vi "Convert Experiment Folder.vi"(8 "error in (no error)":errorcluster, 10 "Experiment Folder File Type":T1, 11 "Experiment Folder Path":path) -> (0 "error out":errorcluster)   [LabVIEW 2016, in "Conversion.lvclass"]
uses:
  Conversion.lvclass
  Data/Typedefs/File Type--enum.ctl
  <userlib>/_OpenG.lib/lvzip/lvzip.llb/ZLIB Zip Handle__ogtk.ctl
  Conversion.lvclass/Conversion.ctl
  <userlib>/_OpenG.lib/file/file.llb/Build Path - File Names Array__ogtk.vi
  <userlib>/_OpenG.lib/file/file.llb/Convert File Extension (Path)__ogtk.vi
  <userlib>/_OpenG.lib/file/file.llb/Compare Two Paths - Scalar__ogtk.vi
  <userlib>/_OpenG.lib/lvzip/lvzip.llb/ZLIB Store File__ogtk.vi
  Data/Data.lvclass
panel:
  out "File":string
  out "State":string
  in  "OK":bool
  in  "Additional Notes?":string
  out "Elapsed Time (s)":dbl
  out "Remaining Files":i32
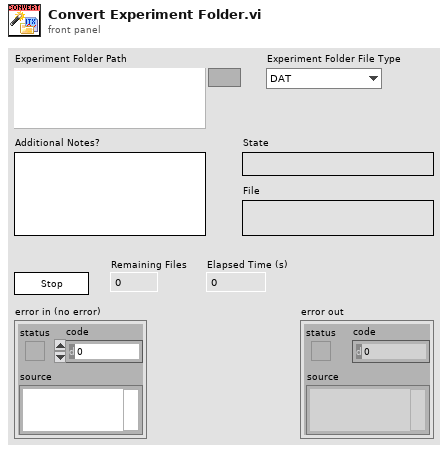
[diagram p1: front panel]
types:
  T1 = typedef "Data.lvclass/File Type--enum.ctl" = enum16{"DAT", "ITX", "TDMS", "VI", "PGSQL"}
  T2 = enum32{"Invalid", "Standard", "Closed", "Hidden", "Minimized", "Maximized"}
  T3 = enum32{"invalid app kind", "Development System", "Run Time System", "Student Edition", "Embedded LabVIEW", "Evaluation", "Custom"}
  T4 = typedef "ZLIB Zip Handle__ogtk.ctl" = refnum<k1>
  T5 = cluster{"Core":cluster{"Current VI Reference":refnum<vi>, "Close Panel on Exit?":bool}, "Conversion.lvclass":refnum<class "Conversion.lvclass">, "Experiment Folder Path":path, "Files to Zip":path[], "zip Refnum":T4, "Start Time":dbl, "Conversion End Time":dbl, "Archive End Time":dbl, "File Index":i32, "Number of Files":i32, "Log File Path":path}
  T6 = cluster{"Current VI Reference":refnum<vi>, "Close Panel on Exit?":bool}
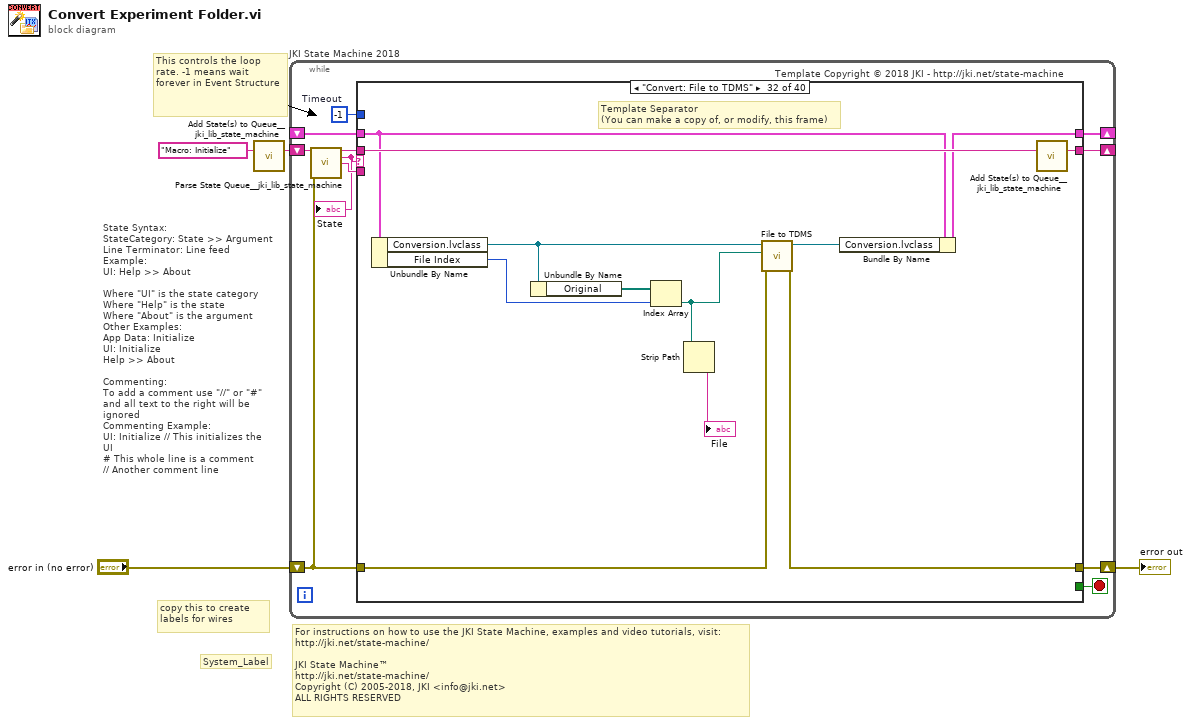
[diagram p0: block diagram]
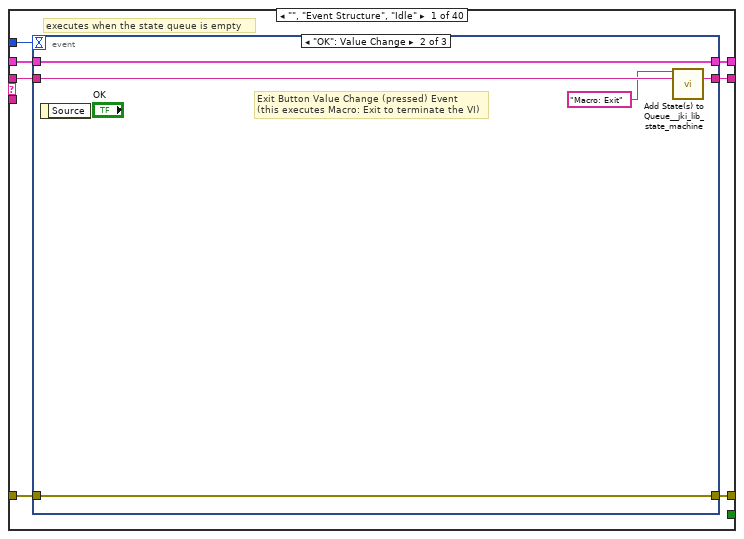
[diagram p2: hidden frame]
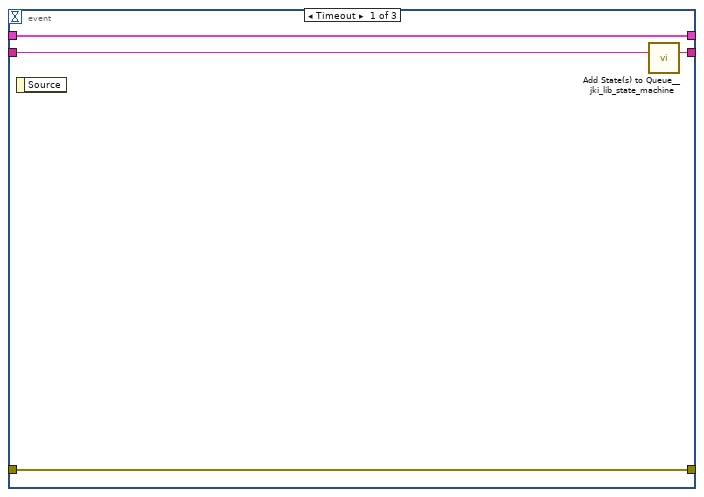
[diagram p3: hidden frame]
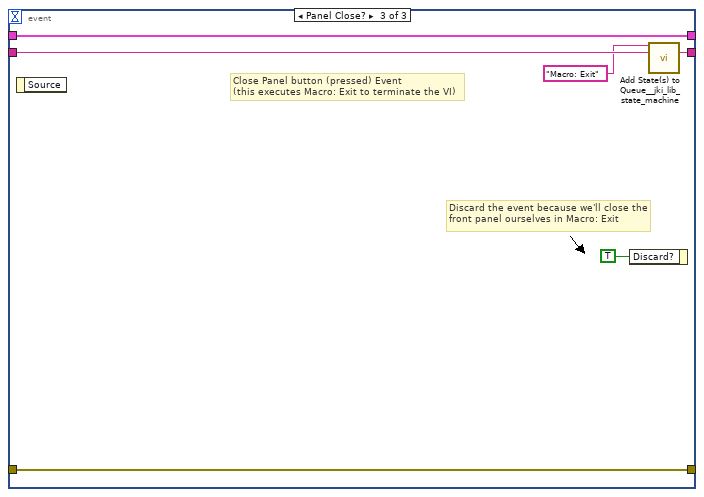
[diagram p4: hidden frame]
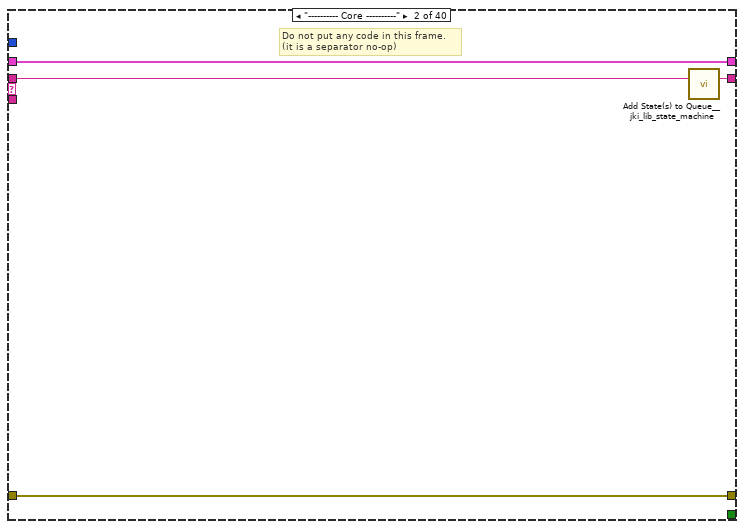
[diagram p5: hidden frame]
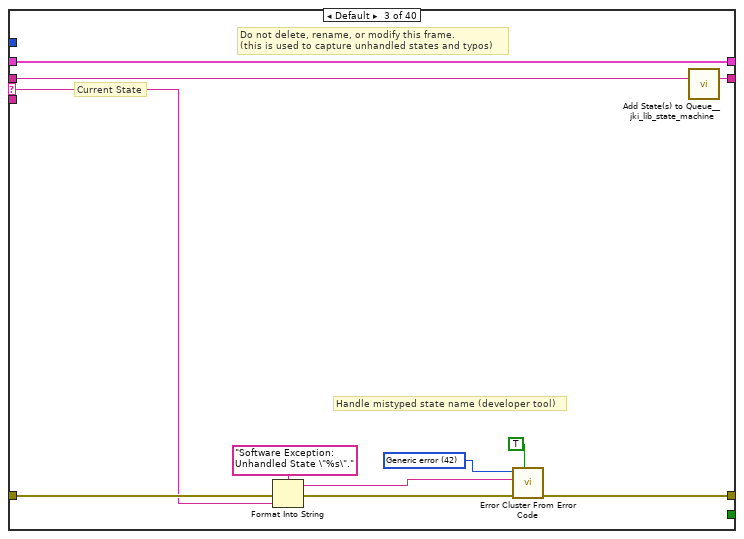
[diagram p6: hidden frame]
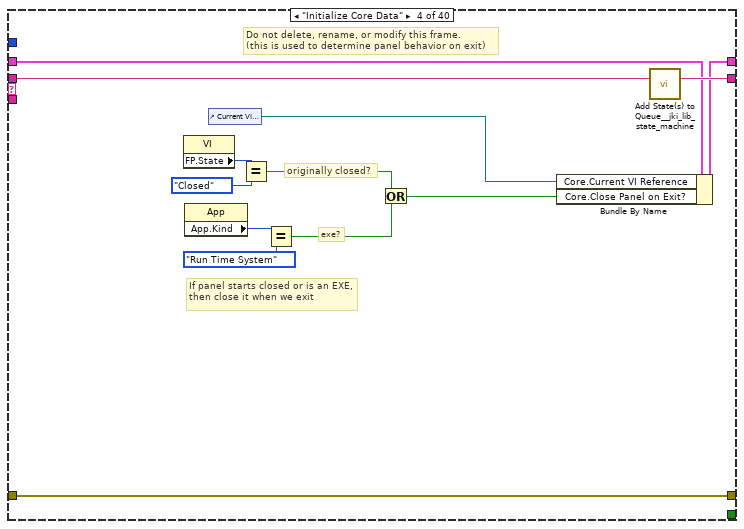
[diagram p7: hidden frame]
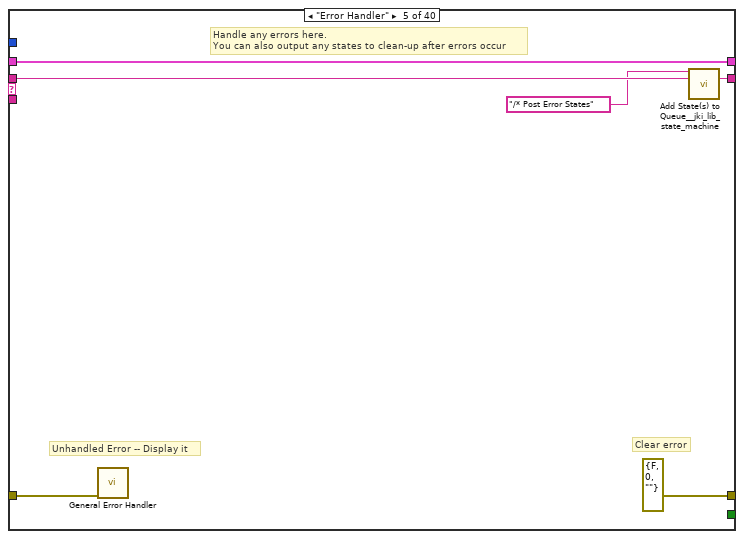
[diagram p8: hidden frame]
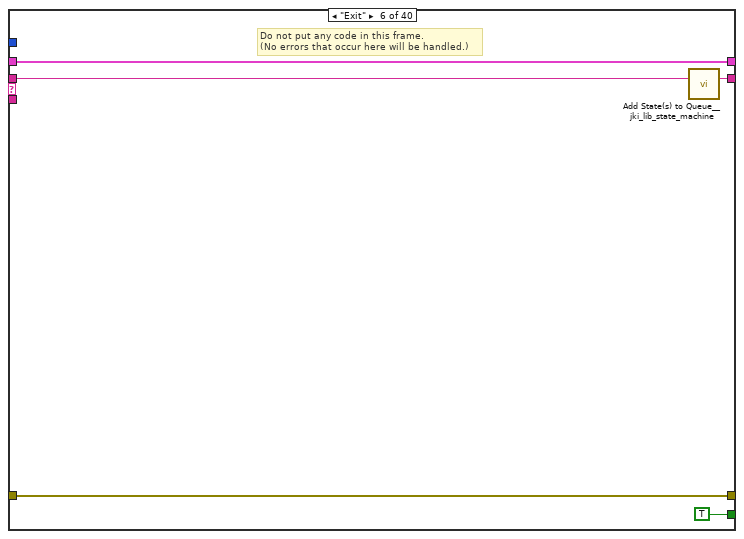
[diagram p9: hidden frame]
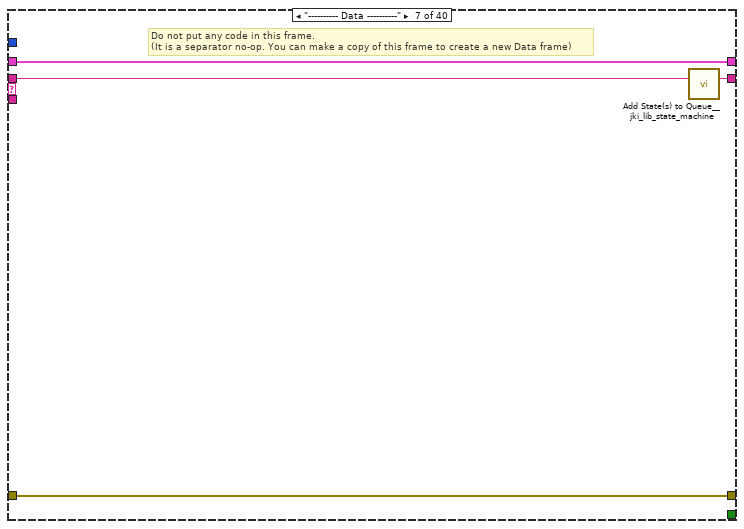
[diagram p10: hidden frame]
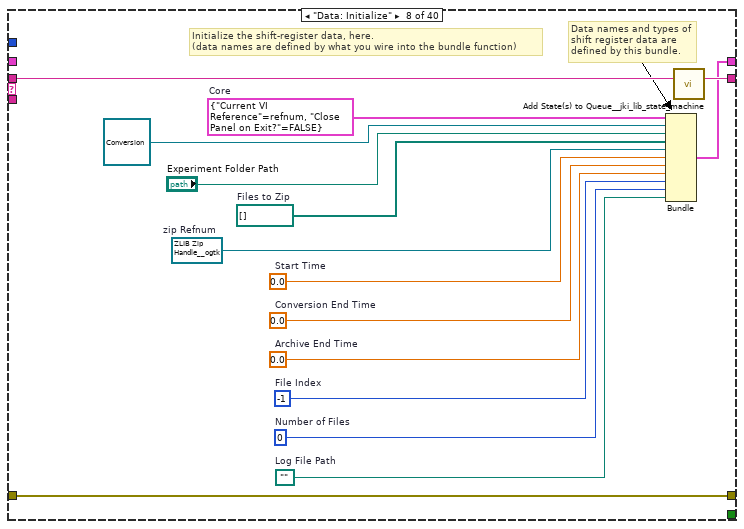
[diagram p11: hidden frame]
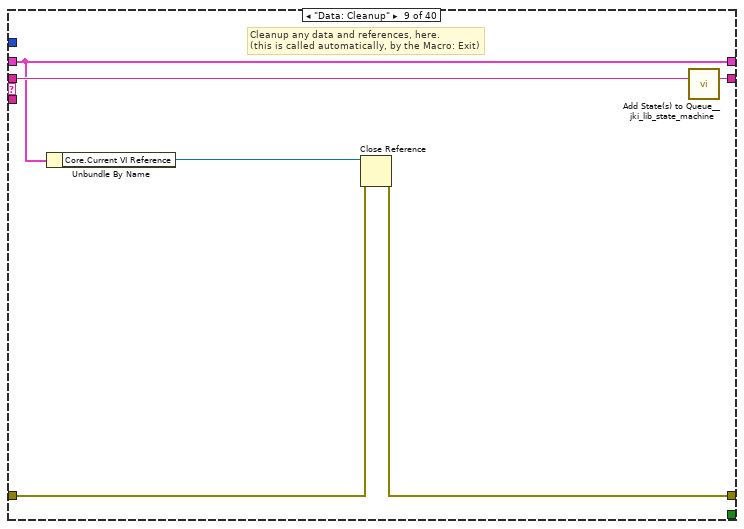
[diagram p12: hidden frame]
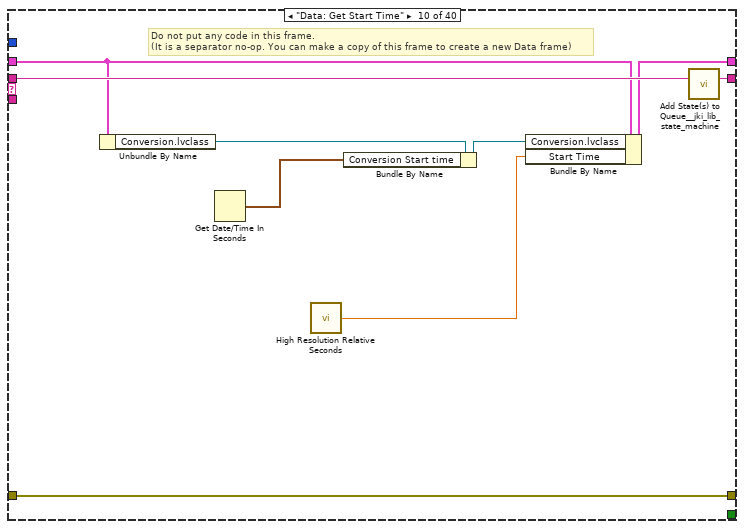
[diagram p13: hidden frame]
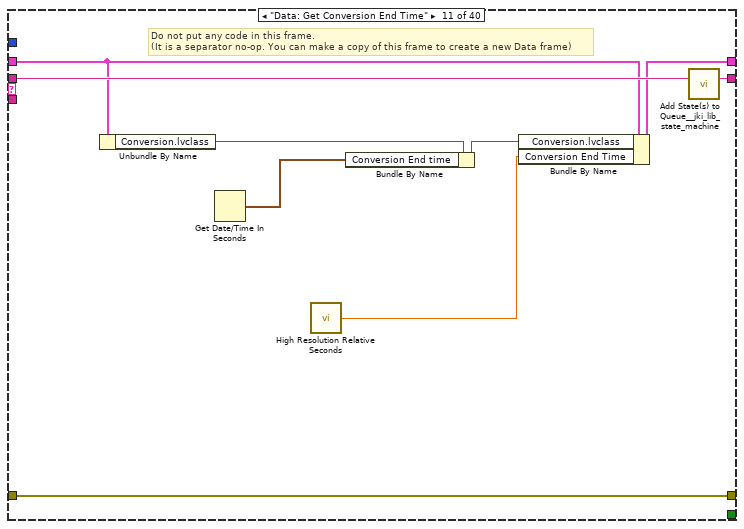
[diagram p14: hidden frame]
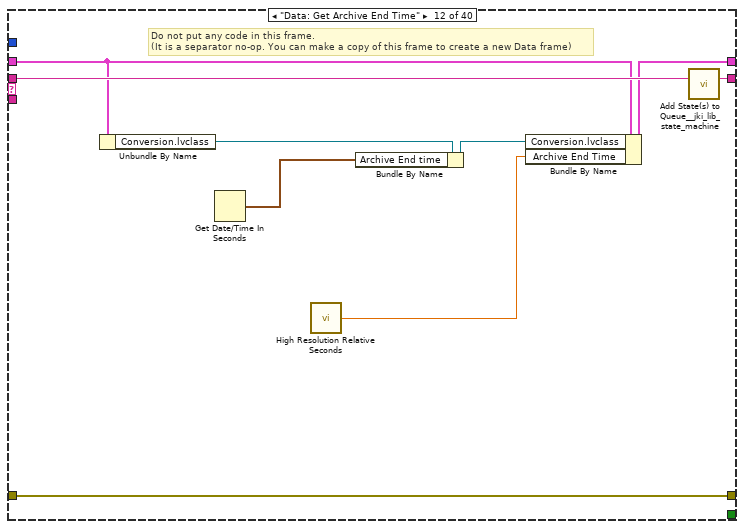
[diagram p15: hidden frame]
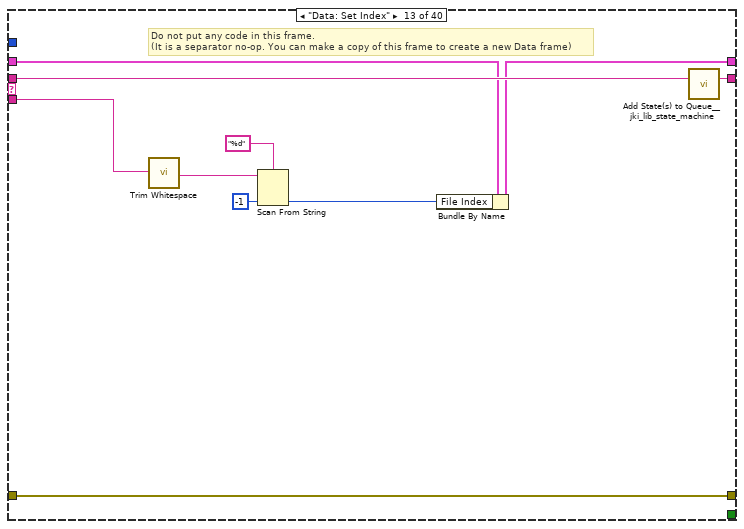
[diagram p16: hidden frame]
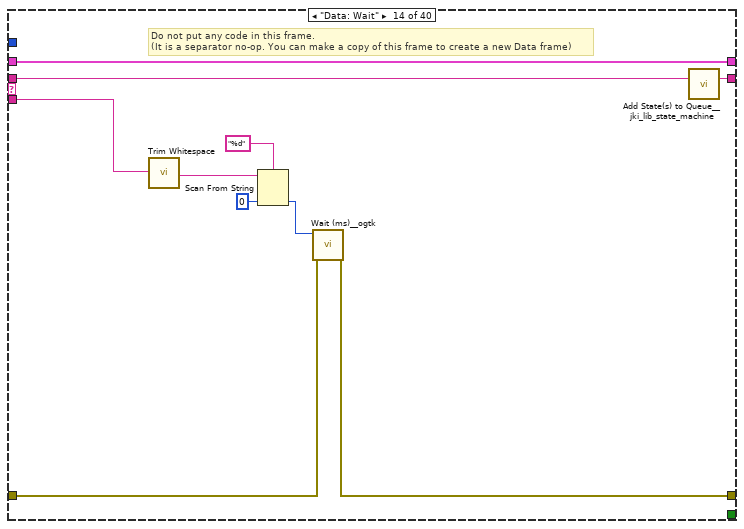
[diagram p17: hidden frame]
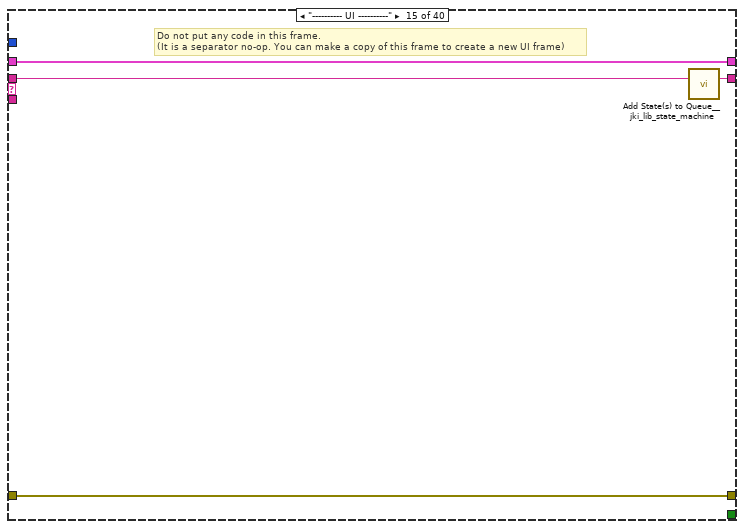
[diagram p18: hidden frame]
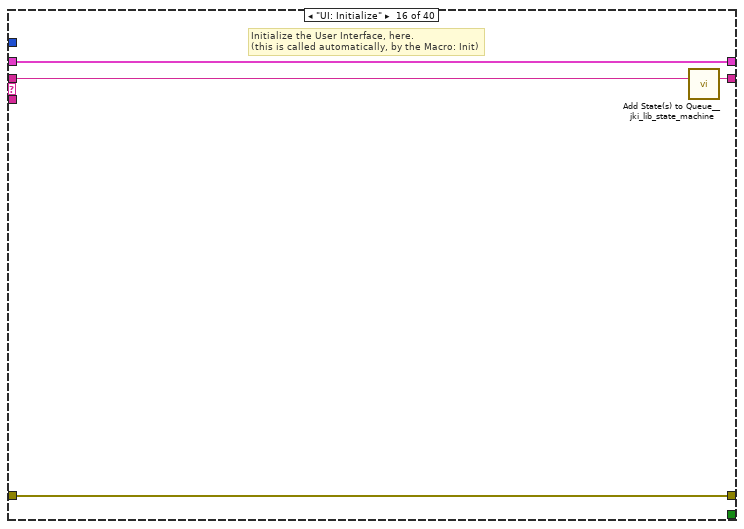
[diagram p19: hidden frame]
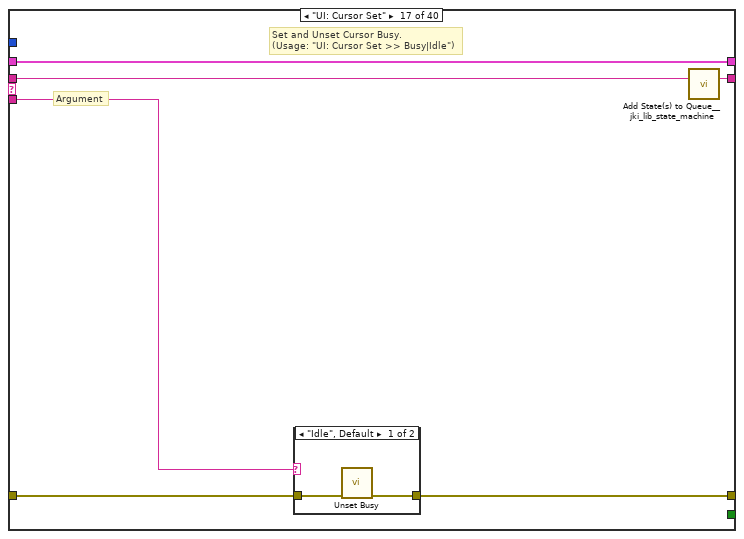
[diagram p20: hidden frame]
diagram:
  # "For instructions on how to use the JKI State Machine, examples and video tutorials, visit:\nhttp://jki.net/state-machine/\n\nJKI State Machine™\nhttp://jki.net/state-machine/\nCopyright (C) 2005-2018, JKI <info@jki.net>\nALL RIGHTS RESERVED"
  # "State Syntax:\nStateCategory: State >> Argument\nLine Terminator: Line feed\nExample:\nUI: Help >> About\n\nWhere \"UI\" is the state category\nWhere \"Help\" is the state\nWhere \"About\" is the argument\nOther Examples:\nApp Data: Initialize\nUI: Initialize\nHelp >> About\n\nCommenting:\nTo add a comment use \"//\" or \"#\" and all text to the right will be ignored\nCommenting Example:\nUI: Initialize // This initializes the UI\n# This whole line is a comment\n// Another comment line"
  # "copy this to create labels for wires"
  # "This controls the loop rate. -1 means wait forever in Event Structure"
  # "System_Label"
  n1 = call <vilib>:"Add State(s) to Queue__jki_lib_state_machine.vi"("State(s) in (\"\")"="Macro: Initialize") -> ("States Out"=w4:string)  [unwired: 14 in]
  n2 = while "JKI State Machine 2018" {
    shift-right: [w9] -> _
    shift-left: _ -> [w8]
    shift-right: [w12] -> w1
    shift-left: "error in (no error)" -> [w6]
    shift-right: [w11] -> _
    shift-left: w4 -> [w13]
    stop <- w10 stop-if-true
    w7 = -1  # Timeout
    # "Template Copyright © 2018 JKI - http://jki.net/state-machine"
    n3 = call <vilib>:"Parse State Queue__jki_lib_state_machine.vi"("State Queue"=w13, "Error In (no error)"=w6) -> ("Remaining States"=w15:string, "Current State"=w5:string, "Arguments"=w14:string)  [unwired: 11 in]
    "State" <- w5
    n4 = case shown="\"Convert: File to TDMS\"" w5 {
      selector: w5 -> [_ _ w42 _ _ _ _ _ _ _ _ _ _ _ _ _ _ _ _ _ _ _ _ _ _ _ _ _ _ _ _ _ _ _ _ _ _ _ _ _]
      tunnel: w15 -> [w22 w41 w46 w65 w71 w76 w80 w95 w101 w110 w119 w128 w138 w148 w152 w156 w162 w173 w245 w252 w256 w261 w266 w282 w287 w292 w307 w312 w322 w326 w341 w356 w368 w375 w385 w396 w401 w420 w437 w443]
      tunnel: w14 -> [_ _ _ _ _ _ _ _ _ _ _ _ w129 w142 _ _ w157 w167 _ _ _ _ _ _ _ _ _ _ _ _ _ _ _ _ _ _ _ _ _ _]
      tunnel: w8 -> [w20 w38 w44 w58 w68 w74 w77 _ w96 w107 w116 w125 w134 w146 w149 w154 w160 w169 w242 w249 w253 w258 w263 w270 w284 w289 w295 w309 w319 w323 w338 w351 w365 w371 w379 w392 w398 w413 w433 w440]
      tunnel: [w19 w39 w48 w62 errorcluster {"status"=FALSE, "code"=0, "source"=""} ("error out") w73 w78 w92 w97 w108 w117 w126 w136 w139 w150 w153 w158 w170 w243 w250 w254 w259 w264 w280 w285 w290 w305 w310 w320 w324 w333 w354 w360 w369 w381 w386 w399 w418 w428 w438] -> w12
      tunnel: w6 -> [w18 w39 w47 w62 w67 w73 w78 w92 w98 w108 w117 w126 w136 w140 w150 w153 w159 w171 w243 w250 w254 w259 w264 w280 w285 w290 w305 w310 w320 w324 w334 w345 w361 w370 w382 w387 w399 w409 w427 w439]
      tunnel: [w21 w40 w45 w64 w70 w75 w79 w94 w100 w109 w118 w127 w137 w147 w151 w155 w161 w172 w244 w251 w255 w260 w265 w281 w286 w291 w306 w311 w321 w325 w340 w355 w367 w374 w384 w395 w400 w419 w436 w442] -> w11
      tunnel: [_ _ _ _ _ TRUE _ _ _ _ _ _ _ _ _ _ _ _ _ _ _ _ _ _ _ _ _ _ _ _ _ _ _ _ _ _ _ _ _ _] -> w10
      tunnel: [w17 w38 w44 w63 w68 w74 w77 w93 w96 w106 w115 w124 w135 w146 w149 w154 w160 w169 w242 w249 w253 w258 w263 w270 w284 w289 w295 w309 w319 w323 w337 w350 w364 w371 w378 w392 w398 w412 w432 w440] -> w9
      tunnel: w7 -> [w16 _ _ _ _ _ _ _ _ _ _ _ _ _ _ _ _ _ _ _ _ _ _ _ _ _ _ _ _ _ _ _ _ _ _ _ _ _ _ _]
      frame "", "Event Structure", "Idle" {
        # "executes when the state queue is empty"
        n5 = event shown="[1] \"OK\": Value Change" {
          selector: _ -> [_ _ _]
          dyn-events: _ -> [_ _ _]
          timeout: w16 -> [_ _ _]
          tunnel: w22 -> [w26 w31 w37]
          tunnel: [w25 w30 w36] -> w21
          tunnel: w20 -> [w24 w28 w34]
          tunnel: [w23 w29 w35] -> w19
          tunnel: w18 -> [w23 w29 w35]
          tunnel: [w24 w28 w34] -> w17
          event Timeout {
            n6 = event-data() -> ()  [unwired: 1 in, 1 out]
            n7 = call <vilib>:"Add State(s) to Queue__jki_lib_state_machine.vi"("State(s) in (\"\")"=w26) -> ("States Out"=w25:string)  [unwired: 14 in]
          }
          event "OK": Value Change {
            # "Exit Button Value Change (pressed) Event\n(this executes Macro: Exit to terminate the VI)"
            n8 = event-data() -> ()  [unwired: 1 in, 1 out]
            n9 = call <vilib>:"Add State(s) to Queue__jki_lib_state_machine.vi"("State(s) in Front (\"\")"="Macro: Exit", "State(s) in (\"\")"=w31) -> ("States Out"=w30:string)  [unwired: 13 in]
          }
          event Panel Close? {
            # "Discard the event because we'll close the front panel ourselves in Macro: Exit"
            # "Close Panel button (pressed) Event\n(this executes Macro: Exit to terminate the VI)"
            n10 = event-data() -> ()  [unwired: 1 in, 1 out]
            n11 = event-data("Discard?"=TRUE) -> ()  [unwired: 1 in, 1 out]
            n12 = call <vilib>:"Add State(s) to Queue__jki_lib_state_machine.vi"("State(s) in Front (\"\")"="Macro: Exit", "State(s) in (\"\")"=w37) -> ("States Out"=w36:string)  [unwired: 13 in]
          }
        }
      }
      frame "---------- Core ----------" {
        # "Do not put any code in this frame.\n(it is a separator no-op)"
        n13 = call <vilib>:"Add State(s) to Queue__jki_lib_state_machine.vi"("State(s) in (\"\")"=w41) -> ("States Out"=w40:string)  [unwired: 14 in]
      }
      frame Default {
        w51 = 42 items=["No error", "Argument error", "Memory is full", "Out of zone", "End of file", "File already open", "Generic file I/O error", "File not found", "File permission error", "Disk is full", "Duplicate path", "Too many files open", "System feature not enabled", "Resource file not found", "Cannot add resource", "Resource not found", "Image not found", "Image memory error", "Pen does not exist", "Config type invalid", "Config token not found", "Config parse error", "Config memory error", "Bad external code format", "Bad external code offset", "External code not present", "Null window", "Destroy window error", "Null menu", "Print aborted", "Bad print record", "Print driver error", "Windows error during printing", "Memory error during printing", "Print dialog error", "Generic print error", "Invalid device refnum", "Device not found", "Device parameter error", "Device unit error", "Cannot open device", "Device call aborted", "Generic error", "Cancelled by user", "Object ID too low", "Object ID too high", "Object not in heap", "Unknown heap", "Unknown object (invalid DefProc)", "Unknown object (DefProc not in table)", "Message out of range", "Invalid (null) method", "Unknown message", "Manager call not supported", "Bad address", "Network operation in progress", "Network operation timed out", "Connection is busy", "Network attribute not supported", "Network error", "Address in use", "System out of memory", "Connection aborted", "Connection refused", "Not connected", "Already connected", "Connection closed", "Initialization error (interapplication manager)", "Bad occurrence", "Wait on unbound occurrence handler", "Occurrence queue overflow", "Datalog type conflict", "Unused", "Unrecognized type (interapplication manager)", "Memory corrupt", "Failed to make temporary DLL", "Old CIN version", "Drag socket not found", "Failed to load drop-object", "Failed to register OLE object", "Failed to release OLE object", "Format specifier type mismatch", "Unknown format specifier", "Too few format specifiers", "Too many format specifiers", "Scan failed", "Newer CIN version", "Error converting to variant", "Runtime menu error", "Password tampered", "Variant attribute not found", "Incompatible variant data type", "Event data is not available", "Event Store is not present", "Occurrence is not found", "Event Queue is not created", "Event info is not available", "Refnum passed is NULL", "Error retrieving Class GUID", "Error retrieving CoClass GUID", "Error retrieving TypeLib GUID.", "Bad built application magic bytes.", "Specific driver is different from the specific driver associated with the Logical Name.", "There is no session opened to the class driver.", "Max Error", "MAX - Error with config objects", "MAX - Error loading configuration", "MAX - Group not supported"]
        # "Current State"
        # "Do not delete, rename, or modify this frame.\n(this is used to capture unhandled states and typos)"
        # "Handle mistyped state name (developer tool)"
        n14 = Format Into String(format string="Software Exception: Unhandled State \"%s\"." ("message"), error in=w47, w42) -> (resulting string=w50:string, error out=w49:errorcluster)  [unwired: 1 in]
        n15 = call <vilib>:"Error Cluster From Error Code.vi"("show call chain? (False)"=TRUE, "error in (no error)"=w49, "error message (\"\")"=w50, "error code (0)"=w51) -> ("error out"=w48:errorcluster)  [unwired: 5 in]
        n16 = call <vilib>:"Add State(s) to Queue__jki_lib_state_machine.vi"("State(s) in (\"\")"=w46) -> ("States Out"=w45:string)  [unwired: 14 in]
      }
      frame "Initialize Core Data" {
        # "Do not delete, rename, or modify this frame.\n(this is used to determine panel behavior on exit)"
        # "originally closed?"
        # "exe?"
        # "If panel starts closed or is an EXE, then close it when we exit"
        n17 = property class="VI"() -> ("FP.State"=w55:T2)  [unwired: 2 in, 2 out]
        n18 = property class="App"() -> ("App.Kind"=w61:T3)  [unwired: 2 in, 2 out]
        n19 = control-ref of="Current VI Reference"() -> (w56:refnum<vi>)
        n20 = Equal?(x=w55, y=T2."Closed" ("Front Panel Window:State")) -> (x = y?=w53:bool)
        n21 = Equal?(x=w61, y=T3."Run Time System" ("Application:Kind")) -> (x = y?=w59:bool)
        n22 = Or(x=w53, y=w59) -> (x .or. y?=w57:bool)
        n23 = Bundle By Name(cluster=w58, "Core.Current VI Reference"=w56, "Core.Close Panel on Exit?"=w57) -> (w63:T5)
        n24 = call <vilib>:"Add State(s) to Queue__jki_lib_state_machine.vi"("State(s) in (\"\")"=w65) -> ("States Out"=w64:string)  [unwired: 14 in]
      }
      frame "Error Handler" {
        # "Unhandled Error -- Display it"
        # "Handle any errors here.\nYou can also output any states to clean-up after errors occur"
        # "Clear error"
        n25 = call <vilib>:"General Error Handler.vi"("error in (no error)"=w67) -> ()  [unwired: 10 in, 5 out]
        n26 = call <vilib>:"Add State(s) to Queue__jki_lib_state_machine.vi"("State(s) in Front (\"\")"="/* Post Error States", "State(s) in (\"\")"=w71) -> ("States Out"=w70:string)  [unwired: 13 in]
      }
      frame "Exit" {
        # "Do not put any code in this frame.\n(No errors that occur here will be handled.)"
        n27 = call <vilib>:"Add State(s) to Queue__jki_lib_state_machine.vi"("State(s) in (\"\")"=w76) -> ("States Out"=w75:string)  [unwired: 14 in]
      }
      frame "---------- Data ----------" {
        # "Do not put any code in this frame.\n(It is a separator no-op. You can make a copy of this frame to create a new Data frame)"
        n28 = call <vilib>:"Add State(s) to Queue__jki_lib_state_machine.vi"("State(s) in (\"\")"=w80) -> ("States Out"=w79:string)  [unwired: 14 in]
      }
      frame "Data: Initialize" {
        w81 = path[] []  # Files to Zip
        w82 = T4 refnum items=["zip"]  # zip Refnum
        w85 = 0.0  # Archive End Time
        w86 = path ""  # Log File Path
        w87 = 0  # Number of Files
        w88 = -1  # File Index
        w89 = 0.0  # Conversion End Time
        w90 = 0.0  # Start Time
        w91 = T6 {"Current VI Reference"=refnum, "Close Panel on Exit?"=FALSE}  # Core
        # "Data names and types of shift register data are defined by this bundle."
        # "Initialize the shift-register data, here.\n(data names are defined by what you wire into the bundle function)"
        n29 = Bundle("Core"=w91, "Conversion.lvclass"=refnum<class "Conversion.lvclass"> refnum, "Experiment Folder Path"="Experiment Folder Path", "Files to Zip"=w81, "zip Refnum"=w82, "Start Time"=w90, "Conversion End Time"=w89, "Archive End Time"=w85, "File Index"=w88, "Number of Files"=w87, "Log File Path"=w86) -> (w93:T5)  [unwired: 1 in]
        n30 = call <vilib>:"Add State(s) to Queue__jki_lib_state_machine.vi"("State(s) in (\"\")"=w95) -> ("States Out"=w94:string)  [unwired: 14 in]
      }
      frame "Data: Cleanup" {
        # "Cleanup any data and references, here.\n(this is called automatically, by the Macro: Exit)"
        n31 = Unbundle By Name(w96) -> ("Core.Current VI Reference"=w99:refnum<vi>)
        n32 = Close Reference(reference=w99, error in (no error)=w98) -> (error out=w97:errorcluster)
        n33 = call <vilib>:"Add State(s) to Queue__jki_lib_state_machine.vi"("State(s) in (\"\")"=w101) -> ("States Out"=w100:string)  [unwired: 14 in]
      }
      frame "Data: Get Start Time" {
        # "Do not put any code in this frame.\n(It is a separator no-op. You can make a copy of this frame to create a new Data frame)"
        n34 = Unbundle By Name(w107) -> ("Conversion.lvclass"=w104:refnum<class "Conversion.lvclass">)
        n35 = Get Date/Time In Seconds() -> (seconds since 1Jan1904=w105:timestamp)
        n36 = call <vilib>:"High Resolution Relative Seconds.vi"() -> ("relative seconds"=w102:dbl)
        n37 = Bundle By Name(cluster=w104, "Conversion Start time"=w105) -> (w103:refnum<class "Conversion.lvclass">)
        n38 = Bundle By Name(cluster=w107, "Conversion.lvclass"=w103, "Start Time"=w102) -> (w106:T5)
        n39 = call <vilib>:"Add State(s) to Queue__jki_lib_state_machine.vi"("State(s) in (\"\")"=w110) -> ("States Out"=w109:string)  [unwired: 14 in]
      }
      frame "Data: Get Conversion End Time" {
        # "Do not put any code in this frame.\n(It is a separator no-op. You can make a copy of this frame to create a new Data frame)"
        n40 = Unbundle By Name(w116) -> ("Conversion.lvclass"=w113:refnum<class "Conversion.lvclass">)
        n41 = Get Date/Time In Seconds() -> (seconds since 1Jan1904=w114:timestamp)
        n42 = call <vilib>:"High Resolution Relative Seconds.vi"() -> ("relative seconds"=w111:dbl)
        n43 = Bundle By Name(cluster=w113, "Conversion End time"=w114) -> (w112:refnum<class "Conversion.lvclass">)
        n44 = Bundle By Name(cluster=w116, "Conversion.lvclass"=w112, "Conversion End Time"=w111) -> (w115:T5)
        n45 = call <vilib>:"Add State(s) to Queue__jki_lib_state_machine.vi"("State(s) in (\"\")"=w119) -> ("States Out"=w118:string)  [unwired: 14 in]
      }
      frame "Data: Get Archive End Time" {
        # "Do not put any code in this frame.\n(It is a separator no-op. You can make a copy of this frame to create a new Data frame)"
        n46 = Unbundle By Name(w125) -> ("Conversion.lvclass"=w122:refnum<class "Conversion.lvclass">)
        n47 = Get Date/Time In Seconds() -> (seconds since 1Jan1904=w123:timestamp)
        n48 = call <vilib>:"High Resolution Relative Seconds.vi"() -> ("relative seconds"=w120:dbl)
        n49 = Bundle By Name(cluster=w122, "Archive End time"=w123) -> (w121:refnum<class "Conversion.lvclass">)
        n50 = Bundle By Name(cluster=w125, "Conversion.lvclass"=w121, "Archive End Time"=w120) -> (w124:T5)
        n51 = call <vilib>:"Add State(s) to Queue__jki_lib_state_machine.vi"("State(s) in (\"\")"=w128) -> ("States Out"=w127:string)  [unwired: 14 in]
      }
      frame "Data: Set Index" {
        # "Do not put any code in this frame.\n(It is a separator no-op. You can make a copy of this frame to create a new Data frame)"
        n52 = call <vilib>:"Trim Whitespace.vi"("string"=w129) -> ("trimmed string"=w133:string)  [unwired: 1 in]
        n53 = Scan From String(format string="%d", input string=w133, default 1=-1 ("default value 1")) -> (output 1=w130:i32)  [unwired: 2 in, 3 out]
        n54 = Bundle By Name(cluster=w134, "File Index"=w130) -> (w135:T5)
        n55 = call <vilib>:"Add State(s) to Queue__jki_lib_state_machine.vi"("State(s) in (\"\")"=w138) -> ("States Out"=w137:string)  [unwired: 14 in]
      }
      frame "Data: Wait" {
        # "Do not put any code in this frame.\n(It is a separator no-op. You can make a copy of this frame to create a new Data frame)"
        n56 = call <vilib>:"Trim Whitespace.vi"("string"=w142) -> ("trimmed string"=w145:string)  [unwired: 1 in]
        n57 = Scan From String(format string="%d", input string=w145, default 1=0 ("default value 1")) -> (output 1=w141:i32)  [unwired: 2 in, 3 out]
        n58 = call <userlib>:"Wait (ms)__ogtk.vi"("error in (no error)"=w140, "milliseconds to wait"=w141) -> ("error out"=w139:errorcluster)  [unwired: 8 in, 1 out]
        n59 = call <vilib>:"Add State(s) to Queue__jki_lib_state_machine.vi"("State(s) in (\"\")"=w148) -> ("States Out"=w147:string)  [unwired: 14 in]
      }
      frame "---------- UI ----------" {
        # "Do not put any code in this frame.\n(It is a separator no-op. You can make a copy of this frame to create a new UI frame)"
        n60 = call <vilib>:"Add State(s) to Queue__jki_lib_state_machine.vi"("State(s) in (\"\")"=w152) -> ("States Out"=w151:string)  [unwired: 14 in]
      }
      frame "UI: Initialize" {
        # "Initialize the User Interface, here.\n(this is called automatically, by the Macro: Init)"
        n61 = call <vilib>:"Add State(s) to Queue__jki_lib_state_machine.vi"("State(s) in (\"\")"=w156) -> ("States Out"=w155:string)  [unwired: 14 in]
      }
      frame "UI: Cursor Set" {
        # "Argument"
        # "Set and Unset Cursor Busy.\n(Usage: \"UI: Cursor Set >> Busy|Idle\")"
        n62 = case shown="\"Idle\", Default" w157 {
          tunnel: w159 -> [w164 w166]
          tunnel: [w163 w165] -> w158
          frame "Idle", Default {
            n63 = call <vilib>:"Unset Busy.vi"("error in (no error)"=w164) -> ("error out"=w163:errorcluster)  [unwired: 10 in]
          }
          frame "Busy" {
            n64 = call <vilib>:"Set Busy.vi"("error in (no error)"=w166) -> ("error out"=w165:errorcluster)  [unwired: 9 in, 1 out]
          }
        }
        n65 = call <vilib>:"Add State(s) to Queue__jki_lib_state_machine.vi"("State(s) in (\"\")"=w162) -> ("States Out"=w161:string)  [unwired: 14 in]
      }
      frame "UI: Front Panel State" {
        # "Argument"
        # "Set Front Panel Open or Closed\n(Usage: \"UI: Front Panel State >> Open|Close\")"
        n66 = Unbundle By Name(w169) -> ("Core.Current VI Reference"=w168:refnum<vi>)
        n67 = case shown="\"Open\", \"Standard\", Default" w167 {
          tunnel: w171 -> [w179 w194 w205 w218 w231]
          tunnel: [w181 w195 w207 w220 w233] -> w170
          tunnel: w168 -> [w180 w192 w206 w219 w232]
          frame "Open", "Standard", Default {
            w174 = T2."Standard" ("State")
            n68 = property class="VI"(reference=w180, error in=w179) -> (reference out=w177:refnum<vi>, error out=w178:errorcluster, "FP.State"=w176:T2)
            n69 = Not Equal?(x=w176, y=w174) -> (x != y?=w175:bool)
            n70 = case shown="False" w175 {
              tunnel: [w185 w187] -> w181
              tunnel: w178 -> [w184 w187]
              tunnel: w177 -> [w183 _]
              tunnel: w174 -> [w182 _]
              frame True {
                n71 = invoke class="VI" method="FP.Open"(reference=w183, error in=w184, "Activate"=TRUE, "State"=w182) -> (error out=w185:errorcluster)  [unwired: 1 in, 4 out]
              }
              frame False {
              }
            }
          }
          frame "Close", "Closed" {
            n72 = property class="VI"(reference=w192, error in=w194) -> (reference out=w191:refnum<vi>, error out=w193:errorcluster, "FP.State"=w189:T2)
            n73 = Not Equal?(x=w189, y=T2."Closed" ("Front Panel Window:State")) -> (x != y?=w188:bool)
            n74 = case shown="True" w188 {
              tunnel: [w196 w199] -> w195
              tunnel: w193 -> [w196 w198]
              tunnel: w191 -> [_ w197]
              frame False {
              }
              frame True {
                n75 = invoke class="VI" method="FP.Close"(reference=w197, error in=w198) -> (error out=w199:errorcluster)  [unwired: 1 in, 2 out]
              }
            }
          }
          frame "Hidden", "Hide" {
            w200 = T2."Hidden" ("State")
            n76 = property class="VI"(reference=w206, error in=w205) -> (reference out=w203:refnum<vi>, error out=w204:errorcluster, "FP.State"=w202:T2)
            n77 = Not Equal?(x=w202, y=w200) -> (x != y?=w201:bool)
            n78 = case shown="True" w201 {
              tunnel: [w211 w212] -> w207
              tunnel: w204 -> [w210 w212]
              tunnel: w203 -> [w209 _]
              tunnel: w200 -> [w208 _]
              frame True {
                n79 = invoke class="VI" method="FP.Open"(reference=w209, error in=w210, "State"=w208) -> (error out=w211:errorcluster)  [unwired: 2 in, 4 out]
              }
              frame False {
              }
            }
          }
          frame "Minimize", "Minimized" {
            w213 = T2."Minimized" ("State")
            n80 = property class="VI"(reference=w219, error in=w218) -> (reference out=w216:refnum<vi>, error out=w217:errorcluster, "FP.State"=w215:T2)
            n81 = Not Equal?(x=w215, y=w213) -> (x != y?=w214:bool)
            n82 = case shown="True" w214 {
              tunnel: [w224 w225] -> w220
              tunnel: w217 -> [w223 w225]
              tunnel: w216 -> [w222 _]
              tunnel: w213 -> [w221 _]
              frame True {
                n83 = invoke class="VI" method="FP.Open"(reference=w222, error in=w223, "State"=w221) -> (error out=w224:errorcluster)  [unwired: 2 in, 4 out]
              }
              frame False {
              }
            }
          }
          frame "Maximize", "Maximized" {
            w226 = T2."Maximized" ("State")
            n84 = property class="VI"(reference=w232, error in=w231) -> (reference out=w229:refnum<vi>, error out=w230:errorcluster, "FP.State"=w228:T2)
            n85 = Not Equal?(x=w228, y=w226) -> (x != y?=w227:bool)
            n86 = case shown="True" w227 {
              tunnel: [w237 w238] -> w233
              tunnel: w230 -> [w236 w238]
              tunnel: w229 -> [w235 _]
              tunnel: w226 -> [w234 _]
              frame True {
                n87 = invoke class="VI" method="FP.Open"(reference=w235, error in=w236, "State"=w234) -> (error out=w237:errorcluster)  [unwired: 2 in, 4 out]
              }
              frame False {
              }
            }
          }
        }
        n88 = call <vilib>:"Add State(s) to Queue__jki_lib_state_machine.vi"("State(s) in (\"\")"=w173) -> ("States Out"=w172:string)  [unwired: 14 in]
      }
      frame "UI: Update Elapsed Time" {
        # "Do not put any code in this frame.\n(It is a separator no-op. You can make a copy of this frame to create a new UI frame)"
        n89 = Unbundle By Name(w242) -> ("Start Time"=w241:dbl)
        n90 = call <vilib>:"High Resolution Relative Seconds.vi"() -> ("relative seconds"=w240:dbl)
        n91 = Subtract(x=w240, y=w241) -> (x-y=→"Elapsed Time (s)":dbl)
        n92 = call <vilib>:"Add State(s) to Queue__jki_lib_state_machine.vi"("State(s) in (\"\")"=w245) -> ("States Out"=w244:string)  [unwired: 14 in]
      }
      frame "UI: Update Index" {
        # "Do not put any code in this frame.\n(It is a separator no-op. You can make a copy of this frame to create a new UI frame)"
        n93 = Unbundle By Name(w249) -> ("Number of Files"=w248:i32, "File Index"=w247:i32)
        n94 = Subtract(x=w248, y=w247) -> (x-y=→"Remaining Files":i32)
        n95 = call <vilib>:"Add State(s) to Queue__jki_lib_state_machine.vi"("State(s) in (\"\")"=w252) -> ("States Out"=w251:string)  [unwired: 14 in]
      }
      frame "---------- Macro ----------" {
        # "Do not put any code in this frame.\n(It is a separator no-op. You can make a copy of this frame to create a new Macro frame)"
        n96 = call <vilib>:"Add State(s) to Queue__jki_lib_state_machine.vi"("State(s) in (\"\")"=w256) -> ("States Out"=w255:string)  [unwired: 14 in]
      }
      frame "Macro: Initialize" {
        w257 = "Data: Initialize\nInitialize Core Data\nUI: Initialize\nUI: Front Panel State >> Open\nMacro: Convert Initialize\nMacro: Convert\nMacro: Zip Initialize\nMacro: Zip\nConvert: Write Log File\nConvert: Display Error\nMacro: Exit"  # Data: Initialize Initialize Core Data UI: Initialize UI: Front Panel State >> Open Macro: Convert Initialize Macro: Convert Macro: Zip Initialize Macro: Zip Convert: Write Log File Convert: Display Error Macro: Exit
        # "Initialization Macro\n(This is called once, when the VI starts)"
        n97 = call <vilib>:"Add State(s) to Queue__jki_lib_state_machine.vi"("State(s) in Front (\"\")"=w257, "State(s) in (\"\")"=w261) -> ("States Out"=w260:string)  [unwired: 13 in]
      }
      frame "Macro: Convert Initialize" {
        # "Initialization Macro\n(This is called once, when the VI starts)"
        n98 = call <vilib>:"Add State(s) to Queue__jki_lib_state_machine.vi"("State(s) in Front (\"\")"="\nData: Set Index >> -1\nConvert: Get Files\nData: Get Start Time\nUI: Update Index\nUI: Update Elapsed Time", "State(s) in (\"\")"=w266) -> ("States Out"=w265:string)  [unwired: 13 in]
      }
      frame "Macro: Convert" {
        # "Still Running?\n(OR are we done?)"
        # "next step"
        # "Initialization Macro\n(This is called once, when the VI starts)"
        n99 = Unbundle By Name(w270) -> ("File Index"=w274:i32, "Conversion.lvclass"=w269:refnum<class "Conversion.lvclass">)
        n100 = Unbundle By Name(w269) -> ("Original"=w268:path[])
        n101 = Increment(x=w274) -> (x+1=w271:i32)
        n102 = Array Size(array=w268) -> (size(s)=w278:i32)
        n103 = Decrement(x=w278) -> (x-1=w279:i32)
        n104 = In Range and Coerce(upper limit=w279, x=w271, lower limit=0) -> (In Range?=w276:bool)  [unwired: 1 out]
        n105 = Format Into String(format string="Data: Set Index >> %d\nUI: Update Index\nUI: Update Elapsed Time\nConvert: File to TDMS\n//\nMacro: Convert", w271) -> (resulting string=w273:string)  [unwired: 2 in, 1 out]
        n106 = Select(t=w273, s=w276, f="Macro: Convert Cleanup ") -> (s? t:f=w267:string)
        n107 = call <vilib>:"Add State(s) to Queue__jki_lib_state_machine.vi"("State(s) in Front (\"\")"=w267, "State(s) in (\"\")"=w282) -> ("States Out"=w281:string)  [unwired: 13 in]
      }
      frame "Macro: Convert Cleanup" {
        # "Initialization Macro\n(This is called once, when the VI starts)"
        n108 = call <vilib>:"Add State(s) to Queue__jki_lib_state_machine.vi"("State(s) in Front (\"\")"="Convert: Close File\nData: Get Conversion End Time\nUI: Update Elapsed Time", "State(s) in (\"\")"=w287) -> ("States Out"=w286:string)  [unwired: 13 in]
      }
      frame "Macro: Zip Initialize" {
        # "Do not put any code in this frame.\n(It is a separator no-op. You can make a copy of this frame to create a new Macro frame)"
        n109 = call <vilib>:"Add State(s) to Queue__jki_lib_state_machine.vi"("State(s) in Front (\"\")"="\nData: Set Index >> -1\nZip: Open\nUI: Update Elapsed Time", "State(s) in (\"\")"=w292) -> ("States Out"=w291:string)  [unwired: 13 in]
      }
      frame "Macro: Zip" {
        # "Still Running?\n(OR are we done?)"
        # "next step"
        # "Do not put any code in this frame.\n(It is a separator no-op. You can make a copy of this frame to create a new Macro frame)"
        n110 = Unbundle By Name(w295) -> ("File Index"=w299:i32, "Files to Zip"=w293:path[])
        n111 = Increment(x=w299) -> (x+1=w296:i32)
        n112 = Array Size(array=w293) -> (size(s)=w303:i32)
        n113 = Decrement(x=w303) -> (x-1=w304:i32)
        n114 = In Range and Coerce(upper limit=w304, x=w296, lower limit=0) -> (In Range?=w301:bool)  [unwired: 1 out]
        n115 = Format Into String(format string="Data: Set Index >> %d\nUI: Update Index\nUI: Update Elapsed Time\nZip: Add File\n//\nMacro: Zip", w296) -> (resulting string=w298:string)  [unwired: 2 in, 1 out]
        n116 = Select(t=w298, s=w301, f="Macro: Zip Cleanup") -> (s? t:f=w294:string)
        n117 = call <vilib>:"Add State(s) to Queue__jki_lib_state_machine.vi"("State(s) in Front (\"\")"=w294, "State(s) in (\"\")"=w307) -> ("States Out"=w306:string)  [unwired: 13 in]
      }
      frame "Macro: Zip Cleanup" {
        # "Do not put any code in this frame.\n(It is a separator no-op. You can make a copy of this frame to create a new Macro frame)"
        n118 = call <vilib>:"Add State(s) to Queue__jki_lib_state_machine.vi"("State(s) in Front (\"\")"="Zip: Close\nData: Get Archive End Time\nUI: Update Elapsed Time\nConvert: Write Log File\nConvert: Display Error", "State(s) in (\"\")"=w312) -> ("States Out"=w311:string)  [unwired: 13 in]
      }
      frame "Macro: Exit" {
        # "Exit Macro\n(This is called once, when the VI exits)"
        n119 = Unbundle By Name(w319) -> ("Core.Close Panel on Exit?"=w318:bool)
        n120 = Select(t="UI: Front Panel State >> Close", s=w318, f="") -> (s? t:f=w315:string)
        n121 = call <vilib>:"Add State(s) to Queue__jki_lib_state_machine.vi"("State(s) in (\"\")"=w315, "State(s) at Back (\"\")"="Data: Cleanup\nExit") -> ("States Out"=w313:string)  [unwired: 13 in]
        n122 = call <vilib>:"Add State(s) to Queue__jki_lib_state_machine.vi"("State(s) in Front (\"\")"=w313, "State(s) in (\"\")"=w322) -> ("States Out"=w321:string)  [unwired: 13 in]
      }
      frame "---------- Convert ----------" {
        # "Template Separator\n(You can make a copy of, or modify, this frame)"
        n123 = call <vilib>:"Add State(s) to Queue__jki_lib_state_machine.vi"("State(s) in (\"\")"=w326) -> ("States Out"=w325:string)  [unwired: 14 in]
      }
      frame "Convert: Get Files" {
        # "Your code here.\n(You can make a copy of, or modify, this frame)"
        n124 = Unbundle By Name(w338) -> ("Conversion.lvclass"=w339:refnum<class "Conversion.lvclass">, "Experiment Folder Path"=w328:path)
        n125 = case shown="\"TDMS\"" "Experiment Folder File Type" {
          tunnel: ["*.dat" ("pattern") "*.itx" ("pattern") "*.tdms" ("pattern")] -> w331
          frame "DAT", Default {
          }
          frame "ITX" {
          }
          frame "TDMS" {
          }
        }
        n126 = List Folder(path=w328, pattern=w331, error in=w334) -> (path out=w336:path, filenames=w335:string[], error out=w333:errorcluster)  [unwired: 1 in, 1 out]
        n127 = call-poly <userlib>:"Build Path__ogtk.vi"("name or relative path"=w335, "base path"=w336) -> ("appended path"=w327:path[])
        n128 = Bundle By Name(cluster=w339, "Original"=w327) -> (w330:refnum<class "Conversion.lvclass">)
        n129 = Array Size(array=w327) -> (size(s)=w329:i32)
        n130 = Bundle By Name(cluster=w338, "Conversion.lvclass"=w330, "Number of Files"=w329) -> (w337:T5)
        n131 = call <vilib>:"Add State(s) to Queue__jki_lib_state_machine.vi"("State(s) in (\"\")"=w341) -> ("States Out"=w340:string)  [unwired: 14 in]
      }
      frame "Convert: File to TDMS" {
        # "Template Separator\n(You can make a copy of, or modify, this frame)"
        n132 = Unbundle By Name(w351) -> ("Conversion.lvclass"=w349:refnum<class "Conversion.lvclass">, "File Index"=w348:i32)
        n133 = Unbundle By Name(w349) -> ("Original"=w353:path[])
        n134 = Index Array(array=w353, index=w348) -> (element=w347:path)
        n135 = Strip Path(path=w347) -> (name=→"File":string)  [unwired: 1 out]
        n136 = call "File to TDMS.vi"("error in (no error)"=w345, "Path"=w347, "Conversion.lvclass"=w349) -> ("error out"=w354:errorcluster, "Conversion.lvclass out"=w352:refnum<class "Conversion.lvclass">)  [unwired: 6 in, 1 out]
        n137 = Bundle By Name(cluster=w351, "Conversion.lvclass"=w352) -> (w350:T5)
        n138 = call <vilib>:"Add State(s) to Queue__jki_lib_state_machine.vi"("State(s) in (\"\")"=w356) -> ("States Out"=w355:string)  [unwired: 14 in]
      }
      frame "Convert: File to postgresSQL" {
        # "Template Separator\n(You can make a copy of, or modify, this frame)"
        n139 = Unbundle By Name(w365) -> ("Conversion.lvclass"=w358:refnum<class "Conversion.lvclass">, "File Index"=w363:i32)
        n140 = Unbundle By Name(w358) -> ("Original"=w366:path[])
        n141 = Index Array(array=w366, index=w363) -> (element=w362:path)
        n142 = Strip Path(path=w362) -> (name=w357:string)  [unwired: 1 out]
        n143 = local write "File"(w357) -> ()
        n144 = call "File to PG.vi"("error in (no error)"=w361, "Path"=w362, "Conversion.lvclass"=w358) -> ("error out"=w360:errorcluster, "Conversion.lvclass out"=w359:refnum<class "Conversion.lvclass">)  [unwired: 6 in, 1 out]
        n145 = Bundle By Name(cluster=w365, "Conversion.lvclass"=w359) -> (w364:T5)
        n146 = call <vilib>:"Add State(s) to Queue__jki_lib_state_machine.vi"("State(s) in (\"\")"=w368) -> ("States Out"=w367:string)  [unwired: 14 in]
      }
      frame "Convert: Close File" {
        # "Template Separator\n(You can make a copy of, or modify, this frame)"
        n147 = Unbundle By Name(w371) -> ("Conversion.lvclass"=w373:refnum<class "Conversion.lvclass">)
        n148 = Unbundle By Name(w373) -> ("Data.lvclass"=w372:refnum<class "Data.lvclass">)
        n149 = call-dynamic "Close.vi"("error in (no error)"=w370, "Data in"=w372) -> ("error out"=w369:errorcluster)  [unwired: 8 in, 1 out]
        n150 = call <vilib>:"Add State(s) to Queue__jki_lib_state_machine.vi"("State(s) in (\"\")"=w375) -> ("States Out"=w374:string)  [unwired: 14 in]
      }
      frame "Convert: Write Log File" {
        # "Your code here.\n(You can make a copy of, or modify, this frame)"
        n151 = Unbundle By Name(w379) -> ("Conversion.lvclass"=w380:refnum<class "Conversion.lvclass">)
        n152 = call "Write Experiment to TDMS Conversion Log.vi"("error in (no error)"=w382, "Additional Notes?"="Additional Notes?", "Conversion.lvclass"=w380) -> ("error out"=w381:errorcluster, "Log File Path"=w376:path, "Conversion.lvclass out"=w377:refnum<class "Conversion.lvclass">)  [unwired: 6 in]
        n153 = Bundle By Name(cluster=w379, "Conversion.lvclass"=w377, "Log File Path"=w376) -> (w378:T5)
        n154 = call <vilib>:"Add State(s) to Queue__jki_lib_state_machine.vi"("State(s) in (\"\")"=w385) -> ("States Out"=w384:string)  [unwired: 14 in]
      }
      frame "Convert: Display Error" {
        # "dialog is shown if errors detected"
        # "Template Separator\n(You can make a copy of, or modify, this frame)"
        n155 = Unbundle By Name(w392) -> ("Conversion.lvclass"=w391:refnum<class "Conversion.lvclass">, "Log File Path"=w388:path)
        n156 = Unbundle By Name(w391) -> ("Failed Conversions"=w390:path[])
        n157 = Array Size(array=w390) -> (size(s)=w389:i32)
        n158 = Format Into String(format string="There was an issue with the file conversoin\nCheck the log file for details:\n%s", error in=w387, w388) -> (resulting string=w393:string, error out=w386:errorcluster)  [unwired: 1 in]
        n159 = case shown="Default" w389 {
          tunnel: w393 -> [_ w397]
          frame 0 {
          }
          frame Default {
            n160 = One Button Dialog(message=w397) -> ()  [unwired: 1 in, 1 out]
          }
        }
        n161 = call <vilib>:"Add State(s) to Queue__jki_lib_state_machine.vi"("State(s) in (\"\")"=w396) -> ("States Out"=w395:string)  [unwired: 14 in]
      }
      frame "---------- Zip ----------" {
        # "Template Separator\n(You can make a copy of, or modify, this frame)"
        n162 = call <vilib>:"Add State(s) to Queue__jki_lib_state_machine.vi"("State(s) in (\"\")"=w401) -> ("States Out"=w400:string)  [unwired: 14 in]
      }
      frame "Zip: Open" {
        # "Template Separator\n(You can make a copy of, or modify, this frame)"
        n163 = Unbundle By Name(w413) -> ("Conversion.lvclass"=w407:refnum<class "Conversion.lvclass">, "Experiment Folder Path"=w414:path)
        n164 = List Folder(path=w414, error in=w409) -> (path out=w416:path, filenames=w415:string[], error out=w410:errorcluster)  [unwired: 2 in, 1 out]
        n165 = Unbundle By Name(w407) -> ("Converted"=w404:path[])
        n166 = for {
          tunnel: w416 -> [w423]
          tunnel: w415 -> [w422] mode=indexing
          tunnel: [w421] -> w406 mode=indexing
          n167 = Build Path(base path=w423, name or relative path=w422) -> (appended path=w421:path)
        }
        n168 = call-poly <userlib>:"Convert File Extension__ogtk.vi"("new ending (none)"="zip" ("Format String"), "file name"=w414) -> ("new filename"=w402:path)  [unwired: 1 out]
        n169 = Build Array (concatenate)(w404, w402) -> (w403:path[])
        n170 = Bundle By Name(cluster=w407, "Converted"=w403) -> (w408:refnum<class "Conversion.lvclass">)
        n171 = Array Size(array=w406) -> (size(s)=w405:i32)
        n172 = call <userlib>:"ZLIB Open Zip Archive__ogtk.vi"("error in (no error)"=w410, "archive name"=w402) -> ("error out"=w418:errorcluster, "zip Refnum"=w411:T4)  [unwired: 3 in, 1 out]
        n173 = Bundle By Name(cluster=w413, "Conversion.lvclass"=w408, "Number of Files"=w405, "Files to Zip"=w406, "zip Refnum"=w411) -> (w412:T5)
        n174 = call <vilib>:"Add State(s) to Queue__jki_lib_state_machine.vi"("State(s) in (\"\")"=w420) -> ("States Out"=w419:string)  [unwired: 14 in]
      }
      frame "Zip: Add File" {
        # "Template Separator\n(You can make a copy of, or modify, this frame)"
        n175 = Unbundle By Name(w433) -> ("zip Refnum"=w435:T4, "Experiment Folder Path"=w426:path, "Files to Zip"=w429:path[], "File Index"=w434:i32)
        n176 = Index Array(array=w429, index=w434) -> (element=w425:path)
        n177 = call-poly <userlib>:"Compare Two Paths__ogtk.vi"("path2"=w425, "path1"=w426) -> ("relative path from 1 to 2"=w430:path)  [unwired: 1 in, 2 out]
        n178 = Strip Path(path=w425) -> (name=w424:string)  [unwired: 1 out]
        n179 = call-poly <userlib>:"ZLIB Store__ogtk.vi"("error in (no error)"=w427, "internal name (same as source name)"=w430, "source path"=w425, "zip Refnum"=w435) -> ("error out"=w428:errorcluster, "zip Refnum out"=w431:T4)  [unwired: 6 in]
        n180 = local write "File"(w424) -> ()
        n181 = Bundle By Name(cluster=w433, "zip Refnum"=w431) -> (w432:T5)
        n182 = call <vilib>:"Add State(s) to Queue__jki_lib_state_machine.vi"("State(s) in (\"\")"=w437) -> ("States Out"=w436:string)  [unwired: 14 in]
      }
      frame "Zip: Close" {
        # "Template Separator\n(You can make a copy of, or modify, this frame)"
        n183 = Unbundle By Name(w440) -> ("zip Refnum"=w441:T4)
        n184 = call <userlib>:"ZLIB Close Zip Archive__ogtk.vi"("error in (no error)"=w439, "zip Refnum"=w441) -> ("error out"=w438:errorcluster)  [unwired: 4 in, 1 out]
        n185 = call <vilib>:"Add State(s) to Queue__jki_lib_state_machine.vi"("State(s) in (\"\")"=w443) -> ("States Out"=w442:string)  [unwired: 14 in]
      }
    }
  }
  "error out" <- w1
